vi "Set_Field.vi"(6 "Magnet PS":u16(ring) items=["Resistive Magnet", "SCM"], 8 "error in (no error)":errorcluster, 10 "Command_message_in":T2, 11 "Command_queue_in":T1) -> (0 "error out":errorcluster, 2 "Command_message_out":T2, 3 "Command_queue_out":T1)   [LabVIEW 2020]
uses:
  Command_Message.ctl
  Command_Queue.ctl
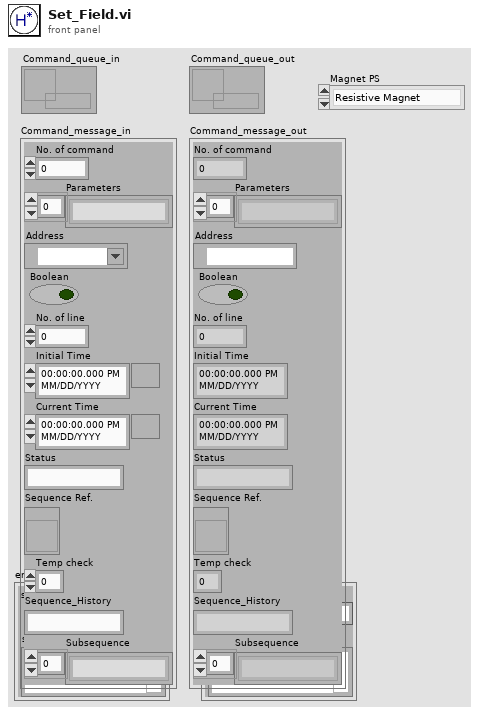
[diagram p1: front panel]
types:
  T1 = typedef "Command_Queue.ctl" = refnum<queue>
  T2 = typedef "Command_Message.ctl" = cluster{"No. of command":i32, "Parameters":string[], "Address":refnum<visa-resource-name>, "Boolean":bool, "No. of line":i32, "Initial Time":timestamp, "Current Time":timestamp, "Status":string, "Sequence Ref.":refnum<vi>, "Temp check":i32, "Sequence_History":string, "Subsequence":string[]}
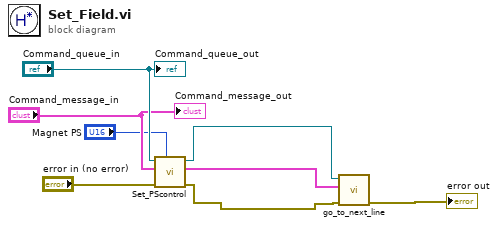
[diagram p0: block diagram]
diagram:
  n1 = call "Set_PScontrol.vi"("Magnet PS"="Magnet PS", "error in (no error)"="error in (no error)", "Command_Message_in"="Command_message_in", "Command_queue_in"="Command_queue_in") -> ("error out"=w1:errorcluster, "Command_Message_out"=w4:T2, "Command_queue_out"=w3:T1)  [unwired: 5 in]
  n2 = call "go_to_next_line.vi"("error in (no error)"=w1, "Message_command in"=w4, "Command Queue in"=w3) -> ("error out"=→"error out":errorcluster)  [unwired: 7 in, 1 out]
  "Command_message_out" <- "Command_message_in"
  "Command_queue_out" <- "Command_queue_in"
